vi "Get Compass Data.vi"(0 "FPGA_MAIN ref in":T1, 5 "error in (no error)":errorcluster) -> (14 "FPGA_MAIN ref out":T1, 16 "Compass Bearing":dbl, 17 "Pitch":dbl, 18 "Roll":dbl, 19 "error out":errorcluster)   [LabVIEW 2009]
uses:
  TypeDefs/Sensor TypeDefs/FPGA Main ref.ctl
  <vilib>/rvi/interface/nirviReadWriteControl/nirviReadWriteControl.xnode
  FPGA Bitfiles/Q_IGVC_2010.lvproj_FPGA Target_FPGA_MAIN.vi.lvbitx
  <vilib>/LabVIEW Targets/FPGA/RIO/nirio_HostInterface/nirio_ReadBig.vi
  <vilib>/rvi/errors/niLvFpgaAdjustHostInterfaceError.vi
  <vilib>/rvi/interface/common/niFpgaNodeNameForErrorReporting.ctl
  <vilib>/rvi/errors/niLvFpgaWhatHappensToTopLevelVI.ctl
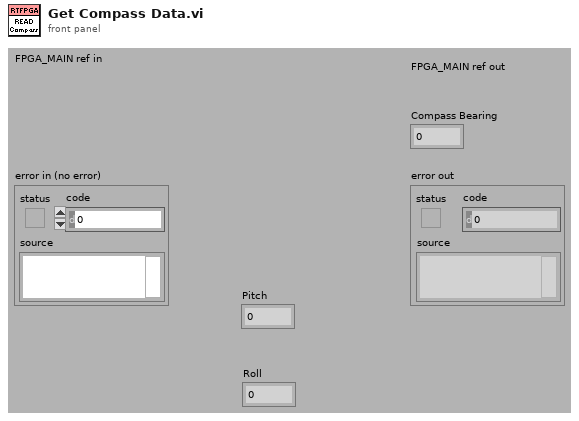
[diagram p1: front panel]
types:
  T1 = typedef "FPGA Main ref.ctl" = refnum<k20>
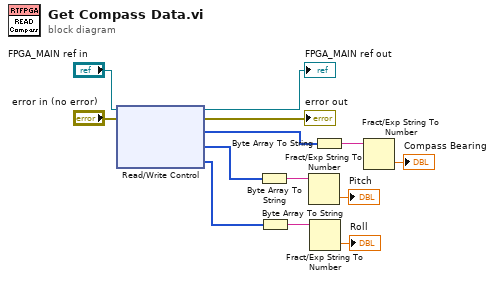
[diagram p0: block diagram]
diagram:
  n1 = xnode "Read/Write Control"("FPGA VI Reference In"="FPGA_MAIN ref in", "error in"="error in (no error)") -> ("FPGA VI Reference Out"=→"FPGA_MAIN ref out":T1, "error out"=→"error out":errorcluster, "heading data"=w11:u8[], "pitch data"=w4:u8[], "roll data"=w1:u8[])
  n2 = Byte Array To String(unsigned byte array=w4) -> (string=w5:string)
  n3 = Byte Array To String(unsigned byte array=w1) -> (string=w3:string)
  n4 = Fract/Exp String To Number(string=w5) -> (number=→"Pitch":dbl)  [unwired: 3 in, 1 out]
  n5 = Fract/Exp String To Number(string=w3) -> (number=→"Roll":dbl)  [unwired: 3 in, 1 out]
  n6 = Byte Array To String(unsigned byte array=w11) -> (string=w10:string)
  n7 = Fract/Exp String To Number(string=w10) -> (number=→"Compass Bearing":dbl)  [unwired: 3 in, 1 out]
